vi "Write Headers.vi"(8 "error in (no error)":errorcluster, 9 "Header Values":string[](array[string]), 10 "Header Names":string[](array[string]), 11 "Linked List Definition in":refnum<class "Linked List Definition.lvclass">) -> (0 "error out":errorcluster, 3 "Linked List Definition out":refnum<class "Linked List Definition.lvclass">)   [LabVIEW 2019, in "Linked Lists.lvlib" / "Linked List Definition.lvclass"]
uses:
  <vilib>/gpm_packages/@cs/linked-list/Source/Linked List/Linked List Definition/Linked List Definition.lvclass
  <vilib>/gpm_packages/@cs/linked-list/Source/Linked List/Linked List Definition/Linked List Definition.lvclass/Linked List Definition.ctl
  <vilib>/gpm_packages/@cs/linked-list/Source/Linked List/Linked List Header/Linked List Header.lvclass
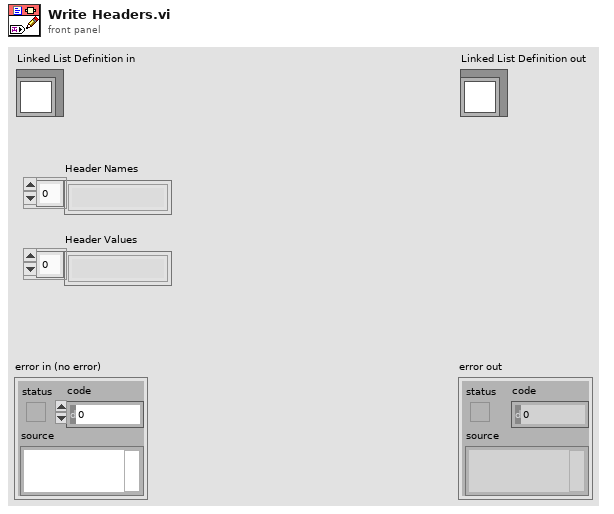
[diagram p1: front panel]
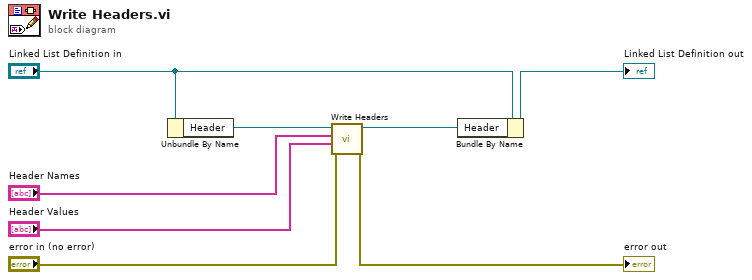
[diagram p0: block diagram]
diagram:
  n1 = Unbundle By Name("Linked List Definition in") -> ("Header"=w8:refnum<class "Linked List Header.lvclass">)
  n2 = call <vilib>:"Write Headers.vi"("error in (no error)"="error in (no error)", "Header Values"="Header Values", "Header Names"="Header Names", "Linked List Header in"=w8) -> ("error out"=→"error out":errorcluster, "Linked List Header out"=w7:refnum<class "Linked List Header.lvclass">)  [unwired: 6 in]
  n3 = Bundle By Name(cluster="Linked List Definition in", "Header"=w7) -> (→"Linked List Definition out":refnum<class "Linked List Definition.lvclass">)
